vi "RatTracker.vi"() -> ()   [LabVIEW 2014]
doc: "Capture_32bit nimmt kontinuierlich Bilder von der Kamera auf und zeigt diese an."
panel:
  out "Elapsed Time (s)":dbl
  out "Rat Name":string
  out "Dropped Frame Count":dbl
  out "AVI Frame Number":dbl
  out "Codec Names":string[](array[string])
  out "error out":errorcluster caption="error"
  out "Video":T1(plugin-control)
  in  "Camera ID":u32
  out "Height":i32=480
  out "Width":i32=640
  out "Bits/Pixel":i32=8
  out "FPS":dbl=6.258409738085552
  in  "Blue Gain":i32(slide) min=0 max=100 scale=0.0..100.0
  in  "Red Gain":i32(slide) min=0 max=100 scale=0.0..100.0
  in  "Green Gain":i32(slide) min=0 max=100 scale=0.0..100.0
  in  "Exposure time":dbl(slide)=33.21525 min=0.0286 max=15.987400000000001 step=0.0286 scale=0.0286..15.987400000000001 scale format="%#.3g"
  in  "Auto Shutter":bool
  in  "Auto Whitebalance":bool
  in  "Color Correction":bool
  in  "Frame rate":dbl(slide)=59.79798117517122 min=1.0506320602474448 max=63.11378152533386 step=2.86e-05 scale=1.0506320602474448..63.11378152533386 scale format="%^#_3g"
  in  "Pixel clock":i32(slide)=29 min=5 max=40 scale=5.0..40.0
  in  "Edge Filter":i32(ring)=2 items=["High"=1, "Low"=2]
  in  "Edge Filter Enable / Disable":bool
  in  "Blacklevel Offset":i32(slide) min=0 max=255 scale=0.0..255.0
  in  "Blacklevel Compensation":bool
  in  "Hotpixel correction":bool
  in  "Master Gain":i32(slide)=90 min=0 max=100 scale=0.0..100.0
  in  "Autogain":bool
  in  "Stop":bool
  # "Hello! Press the white arrow in the top-left to start recording."
  # "NOTE: When ending the program, you must use the STOP button below! Otherwise, you will have to restart the computer in order to use the camera again!"
  # "Stop Program here"
  # "Settings"
  # "Image information"
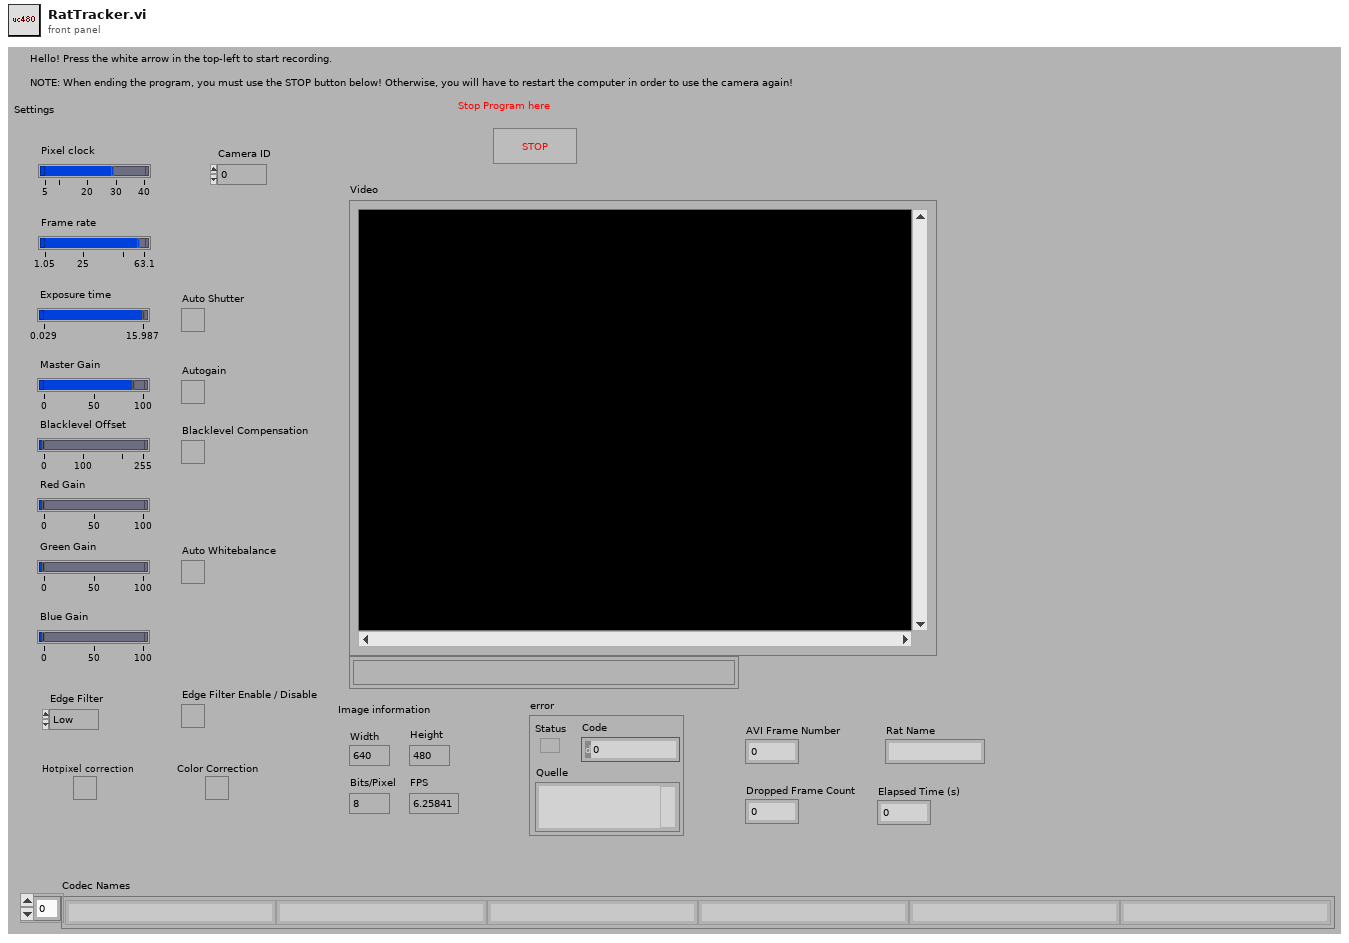
[diagram p1: front panel]
types:
  T1 = typedef "IMAQ Image.ctl" = refnum<image>
  T2 = typedef "IMAQ AVI2 Refnum.ctl" = refnum<k20>
  T3 = cluster{"Height":i32, "Width":i32, "Bits/Pixel":i32}
  T4 = cluster{"Codec Names[0]":string, "Codec Names[1]":string, "Codec Names[2]":string, "Codec Names[3]":string, "Codec Names[4]":string, "Codec Names[5]":string, "Codec Names[6]":string, "Codec Names[7]":string, "Codec Names[8]":string}
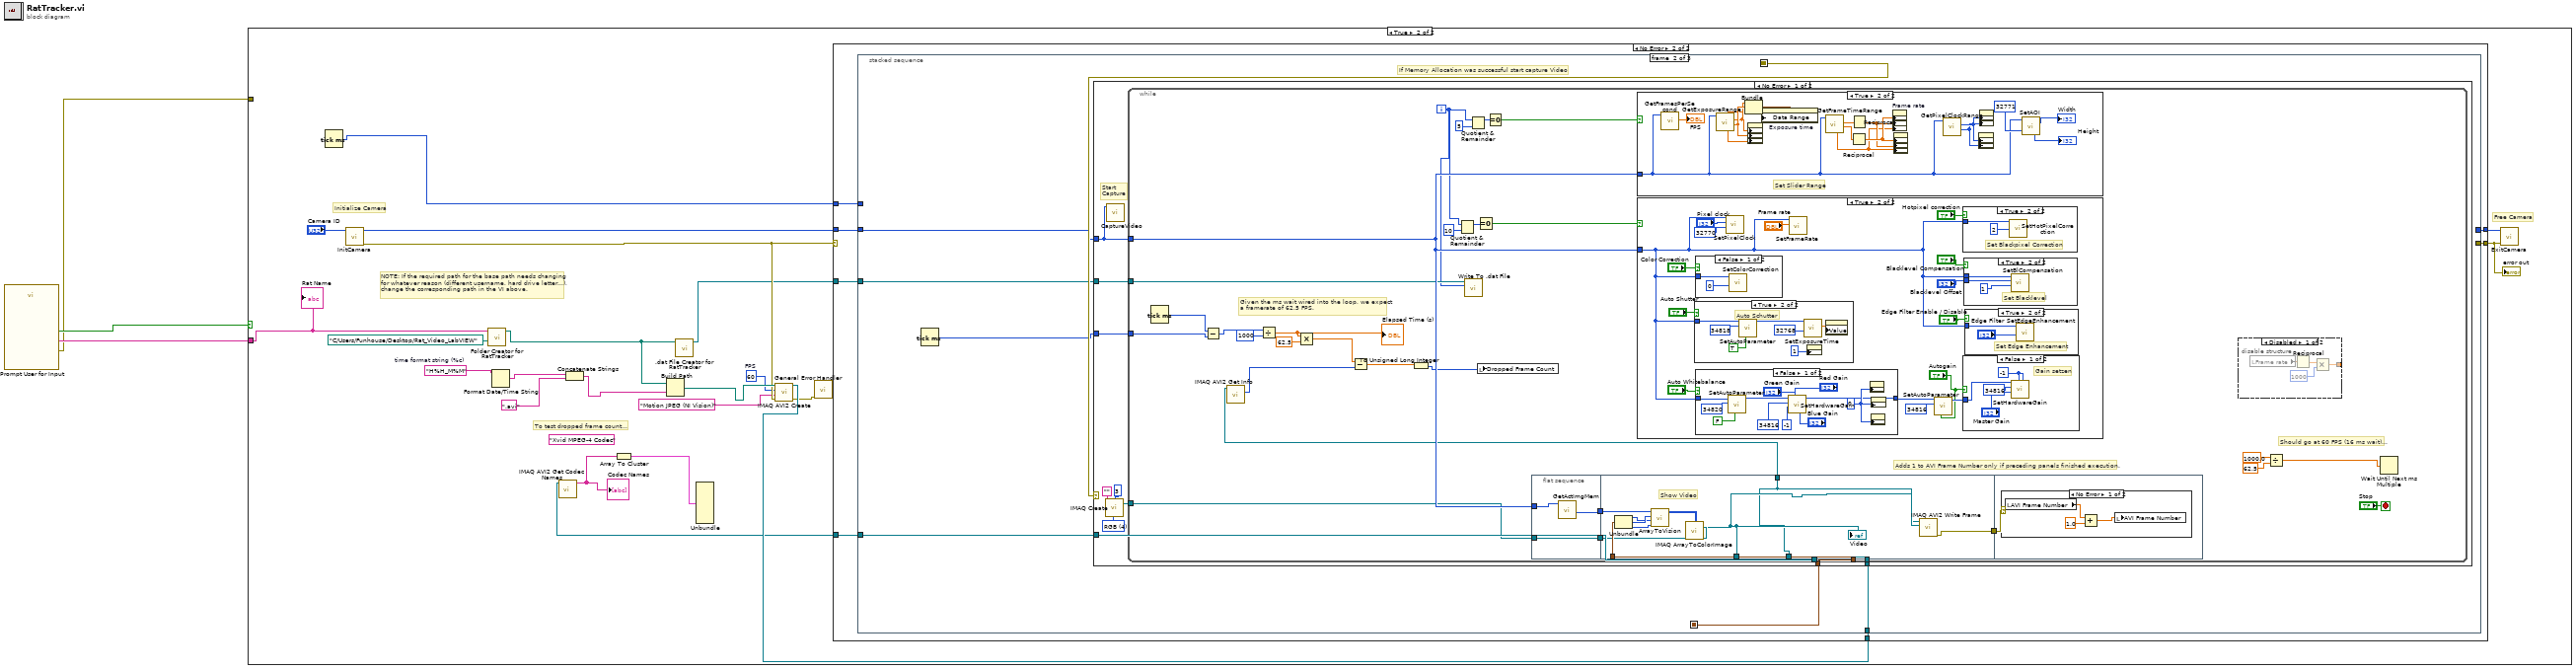
[diagram p0: block diagram]
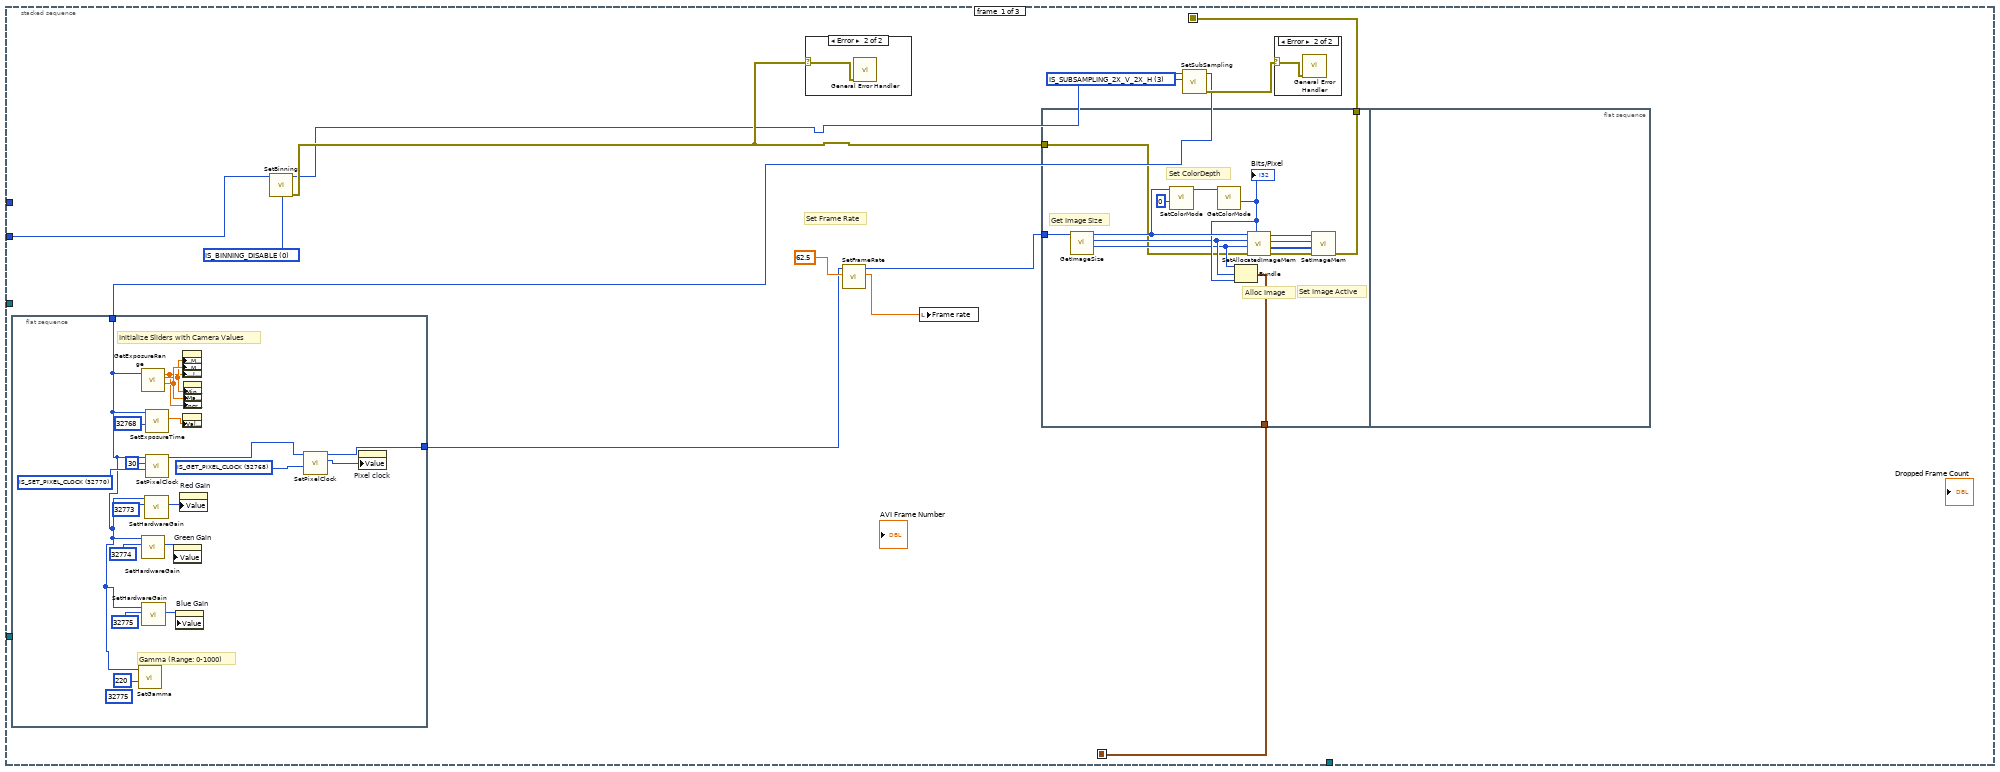
[diagram p4: hidden frame]
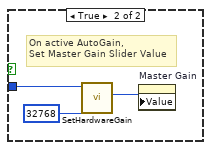
[diagram p9: hidden frame]
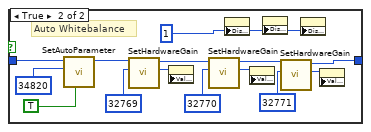
[diagram p10: hidden frame]
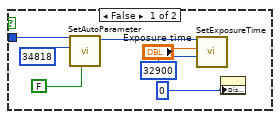
[diagram p11: hidden frame]
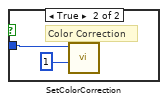
[diagram p12: hidden frame]
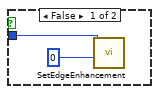
[diagram p13: hidden frame]
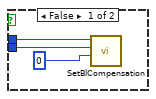
[diagram p14: hidden frame]
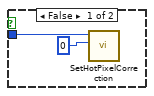
[diagram p15: hidden frame]
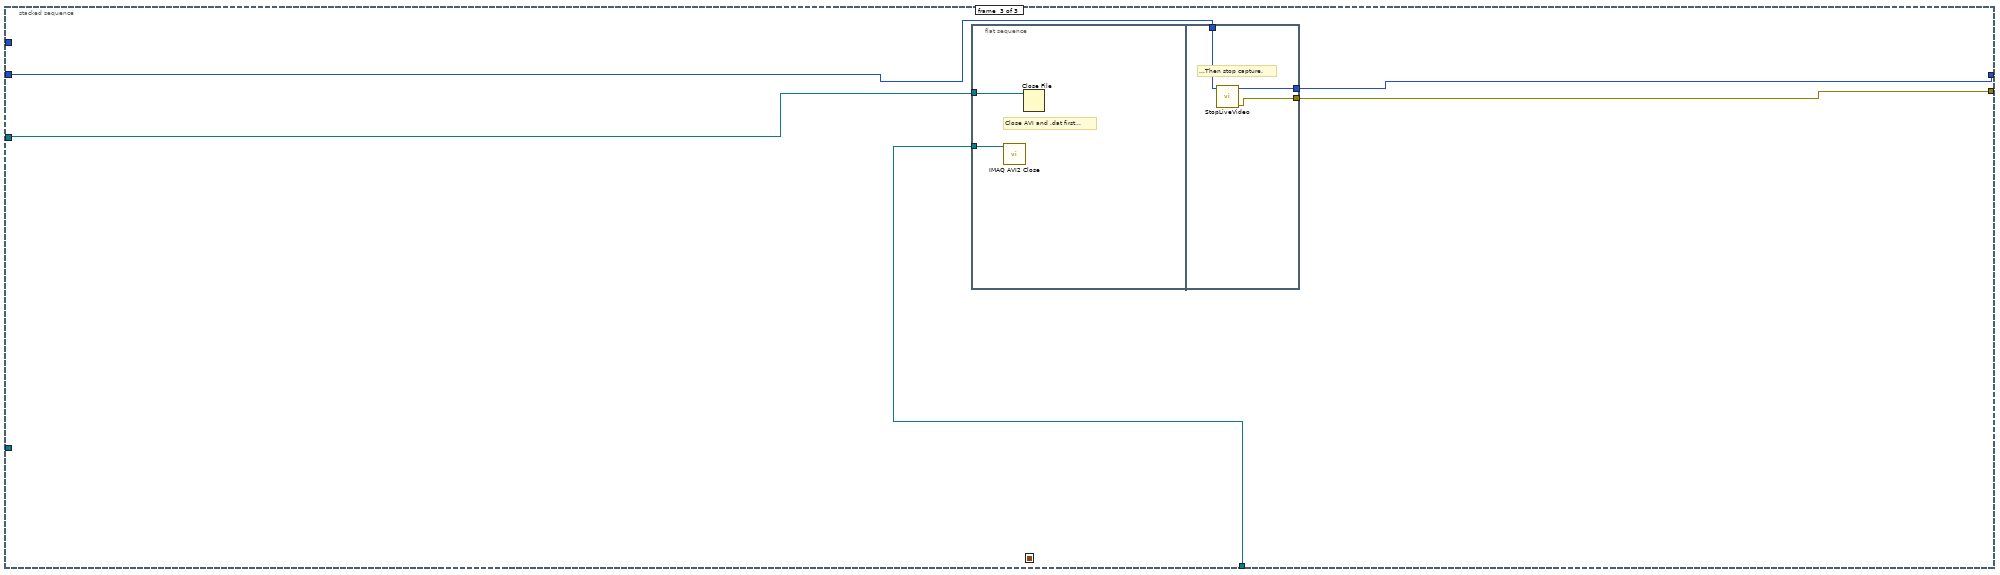
[diagram p19: hidden frame]
diagram:
  n1 = call "Prompt User for Input"() -> ("Name"=w2:string, "OK"=w3:bool, "error out"=w1:errorcluster)  [unwired: 17 in]
  n2 = case shown="True" w3 {
    tunnel: w2 -> [_ w15]
    tunnel: w1 -> [_ _]
    frame False {
    }
    frame True {
      (unwired) "Xvid MPEG-4 Codec"
      w7 = u32 60  # FPS
      w19 = "H%H_M%M"  # time format string (%c)
      # "To test dropped frame count..."
      # "NOTE: If the required path for the base path needs changing\nfor whatever reason (different username, hard drive letter...),\nchange the corresponding path in the VI above."
      # "Free Camera"
      # "Initialize Camera"
      n3 = Tick Count (ms)() -> (millisecond timer value=w5:u32)
      n4 = call "InitCamera.vi"("Camera ID"="Camera ID") -> ("error out"=w12:errorcluster, "Camera Handle Out"=w24:u32)  [unwired: 9 in]
      n5 = call "Folder Creator for RatTracker.vi"("Base Path"=path "C:/Users/Funhouse/Desktop/Rat_Video_LabVIEW" ("Base Path for File"), "Rat Name"=w15) -> ("Path of Folder with .avi and .dat"=w16:path)  [unwired: 9 in]
      n6 = Format Date/Time String(time format string (%c)=w19) -> (date/time string=w20:string)  [unwired: 2 in]
      n7 = Concatenate Strings(w20, ".avi") -> (w17:string)
      n8 = Build Path(base path=w16, name or relative path=w17) -> (appended path=w14:path)
      n9 = call ".dat File Creator for RatTracker.vi"("Path of Folder with .avi and .dat"=w16) -> ("Reference to .dat File"=w8:refnum<file>)  [unwired: 10 in]
      n10 = call "IMAQ AVI2 Create"("error in (no error)"=w12, "Codec"="Motion JPEG (NI Vision)", "Frames Per Second"=w7, "AVI Path"=w14) -> ("error out"=w6:errorcluster, "AVI Refnum"=w13:T2)  [unwired: 6 in]
      n11 = call <vilib>:"General Error Handler.vi"("error in (no error)"=w6) -> ()  [unwired: 10 in, 5 out]
      n12 = case shown="No Error" w12 {
        selector: w12 -> [w26 _]
        tunnel: [w27 w34] -> w25
        tunnel: w24 -> [w27 w33]
        tunnel: [w26 w32] -> w22
        tunnel: w13 -> [_ w31]
        tunnel: [_ w30] -> w11
        tunnel: w8 -> [_ w29]
        tunnel: w5 -> [_ w28]
        frame Error {
        }
        frame No Error {
          n13 = stacked-sequence {
            seq-local: [w46 _ _] -> [_ w89 _]
            seq-local: [w47 _ _] -> [_ w88 _]
            tunnel: w33 -> [w45 w87 w249]
            tunnel: [_ _ w248] -> w34
            tunnel: [_ _ w250] -> w32
            tunnel: w31 -> [_ w86 w251]
            tunnel: [_ w85 _] -> w30
            tunnel: w29 -> [_ w84 w247]
            tunnel: w28 -> [_ _ _]
            frame #0 {
              w40 = 3 items=["IS_SUBSAMPLING_DISABLE"=0, "IS_SUBSAMPLING_2X_V"=1, "IS_SUBSAMPLING_2X_H"=2, "IS_SUBSAMPLING_4X_V"=4, "IS_SUBSAMPLING_4X_H"=8, "IS_SUBSAMPLING_2X_V_2X_H"=3, "IS_SUBSAMPLING_4X_V_2X_H"=6, "IS_SUBSAMPLING_2X_V_4X_H"=9, "IS_SUBSAMPLING_4X_V_4X_H"=12, "IS_GET_SUBSAMPLING"=32768, "IS_GET_SUPPORTED_SUBSAMPLING"=32769] ("Mode")
              w44 = 0 items=["IS_BINNING_DISABLE"=0, "IS_BINNING_2X_V"=1, "IS_BINNING_2X_H"=2, "IS_BINNING_4X_V"=4, "IS_BINNING_4X_H"=8, "IS_BINNING_2X_V_2X_H"=3, "IS_BINNING_2X_V_4X_H"=9, "IS_BINNING_4X_V_2X_H"=6, "IS_BINNING_4X_V_4X_H"=12, "IS_GET_BINNING"=32768, "IS_GET_SUPPORTED_BINNING"=32769] ("Mode")
              # "Set Frame Rate"
              n14 = flat-sequence {
                tunnel: w37 -> [w63]
                tunnel: [w65] -> w36
                frame #0 {
                  (unwired) 32775
                  w68 = 32768 items=["IS_GET_PIXEL_CLOCK"=32768, "IS_GET_DEFAULT_PCLK"=32769, "IS_SET_PIXEL_CLOCK"=32770] ("Mode")
                  w69 = 32770 items=["IS_GET_PIXEL_CLOCK"=32768, "IS_GET_DEFAULT_PCLK"=32769, "IS_SET_PIXEL_CLOCK"=32770] ("Mode")
                  # "Gamma (Range: 0-1000)"
                  # "Initialize Sliders with Camera Values"
                  n15 = call "SetGamma.vi"("Gamma"=220, "Camera Handle In"=w63) -> ()  [unwired: 8 in, 2 out]
                  n16 = call "GetExposureRange.vi"("Camera Handle In"=w63) -> ("max"=w80:dbl, "min"=w79:dbl, "intervall"=w78:dbl)  [unwired: 6 in, 2 out]
                  n17 = call "SetHardwareGain.vi"("Mode"=32774, "Camera Handle In"=w63) -> ("Value"=w73:i32)  [unwired: 7 in, 2 out]
                  n18 = call "SetHardwareGain.vi"("Mode"=32775, "Camera Handle In"=w63) -> ("Value"=w71:i32)  [unwired: 7 in, 2 out]
                  n19 = call "SetHardwareGain.vi"("Mode"=32773, "Camera Handle In"=w63) -> ("Value"=w75:i32)  [unwired: 7 in, 2 out]
                  n20 = call "SetExposureTime.vi"("Mode"=u16 32768, "Camera Handle In"=w63) -> ("new exposure time"=w76:dbl)  [unwired: 7 in, 2 out]
                  n21 = call "SetPixelClock.vi"("Mode"=w69, "Pixel Clock"=30, "Camera Handle In"=w63) -> ("Camera Handle Out"=w67:u32)  [unwired: 6 in, 2 out]
                  n22 = property on="Green Gain" class="Slide (strict)"("Value"=w73) -> ()  [unwired: 2 in, 2 out]
                  n23 = property on="Blue Gain" class="Slide (strict)"("Value"=w71) -> ()  [unwired: 2 in, 2 out]
                  n24 = property on="Red Gain" class="Slide (strict)"("Value"=w75) -> ()  [unwired: 2 in, 2 out]
                  n25 = property on="Exposure time" class="Schieberegler (strikt)"("Scale.Minimum"=w79, "Scale.Maximum"=w80, "Scale.Increment"=w78) -> ()  [unwired: 2 in, 2 out]
                  n26 = property on="Exposure time" class="Schieberegler (strikt)"("Value"=w76) -> ()  [unwired: 2 in, 2 out]
                  n27 = property on="Exposure time" class="Schieberegler (strikt)"("Minimum"=w79, "Maximum"=w80, "Increment"=w78) -> ()  [unwired: 2 in, 2 out]
                  n28 = call "SetPixelClock.vi"("Mode"=w68, "Camera Handle In"=w67) -> ("Value"=w66:i32, "Camera Handle Out"=w65:u32)  [unwired: 7 in, 1 out]
                  n29 = property on="Pixel clock" class="Slide (strict)"("Value"=w66) -> ()  [unwired: 2 in, 2 out]
                }
              }
              n30 = call "SetBinning.vi"("Mode"=w44, "Camera Handle In"=w45) -> ("error out"=w43:errorcluster, "Camera Handle Out"=w42:u32)  [unwired: 7 in, 1 out]
              n31 = case shown="Error" w43 {
                selector: w43 -> [_ w82]
                frame No Error {
                }
                frame Error {
                  n32 = call <vilib>:"General Error Handler.vi"("error in (no error)"=w82) -> ()  [unwired: 10 in, 5 out]
                }
              }
              n33 = call "SetFrameRate.vi"("FPS"=62.5, "Camera Handle In"=w36) -> ("new FPS"=w35:dbl, "Camera Handle Out"=w39:u32)  [unwired: 7 in, 1 out]
              n34 = local write "Frame rate"(w35) -> ()
              n35 = flat-sequence {
                tunnel: [w58] -> w47
                tunnel: [w56] -> w46
                tunnel: w43 -> [w49]
                tunnel: w39 -> [w48]
                frame #0 {
                  # "Set Image Active"
                  # "Alloc Image"
                  # "Set ColorDepth"
                  # "Get Image Size"
                  n36 = call "GetImageSize.vi"("Camera Handle In"=w48) -> ("Height"=w50:i32, "Width"=w51:i32, "Camera Handle Out"=w57:u32)  [unwired: 8 in]
                  n37 = call "SetColorMode.vi"("Mode"=0, "Camera Handle In"=w57) -> ("Camera Handle Out"=w53:u32)  [unwired: 8 in, 1 out]
                  n38 = call "GetColorMode.vi"("Camera Handle In"=w53) -> ("Bits/Pixel"=w52:i32)  [unwired: 8 in, 2 out]
                  "Bits/Pixel" <- w52
                  n39 = Bundle("Height"=w50, "Width"=w51, "Bits/Pixel"=w52) -> (w56:T3)  [unwired: 1 in]
                  n40 = call "SetAllocatedImageMem.vi"("BitsPixel"=w52, "error in"=w49, "Height"=w50, "Width"=w51, "Camera Handle In"=w57) -> ("error out"=w55:errorcluster, "Image Memory Out"=w59:u8[], "Memory ID Out"=w60:i32, "Camera Handle Out"=w61:u32)  [unwired: 2 in, 1 out]
                  n41 = call "SetImageMem.vi"("error in"=w55, "Image Memory In"=w59, "Memory ID In"=w60, "Camera Handle In"=w61) -> ("error out"=w58:errorcluster)  [unwired: 4 in, 3 out]
                }
                frame #1 {
                }
              }
              n42 = call "SetSubSampling.vi"("Mode"=w40, "Camera Handle In"=w42) -> ("error out"=w41:errorcluster, "Camera Handle Out"=w37:u32)  [unwired: 7 in, 1 out]
              n43 = case shown="Error" w41 {
                selector: w41 -> [_ w81]
                frame No Error {
                }
                frame Error {
                  n44 = call <vilib>:"General Error Handler.vi"("error in (no error)"=w81) -> ()  [unwired: 10 in, 5 out]
                }
              }
            }
            frame #1 {
              # "If Memory Allocation was successful start capture Video"
              n45 = Tick Count (ms)() -> (millisecond timer value=w83:u32)
              n46 = case shown="No Error" w88 {
                tunnel: w87 -> [w98 _]
                tunnel: w89 -> [w99 _]
                tunnel: w86 -> [w93 _]
                tunnel: [w92 _] -> w85
                tunnel: w84 -> [w91 _]
                tunnel: w83 -> [w90 _]
                frame No Error {
                  w96 = u32 4 items=["8 bits", "16 bits", "Float", "Complex", "RGB", "HSL"] ("Image Type")
                  # "Start\nCapture"
                  n47 = call "IMAQ Create"("Border Size"=3, "Image Name"="", "Image Type"=w96) -> ("New Image"=w94:T1)  [unwired: 2 in, 1 out]
                  n48 = call "CaptureVideo.vi"("Camera Handle In"=w98) -> ()  [unwired: 9 in, 2 out]
                  n49 = while {
                    tunnel: w99 -> [w129]
                    tunnel: w98 -> [w121]
                    tunnel: w94 -> [w119]
                    tunnel: w93 -> [w118]
                    tunnel: [w117] -> w92
                    tunnel: w91 -> [w116]
                    tunnel: w90 -> [w112]
                    i -> [w115]
                    stop <- "Stop" stop-if-true
                    # "Given the ms wait wired into the loop, we expect\na framerate of 62.5 FPS."
                    # "Should go at 60 FPS (16 ms wait)..."
                    # "Adds 1 to AVI Frame Number only if preceding panels finished execution."
                    n50 = Tick Count (ms)() -> (millisecond timer value=w111:u32)
                    n51 = Subtract(x=w111, y=w112) -> (x-y=w110:u32)
                    n52 = call "IMAQ AVI2 Get Info"("AVI Refnum"=w113) -> ("Number of Frames"=w105:u32)  [unwired: 6 in, 4 out]
                    n53 = Divide(x=w110, y=u32 1000) -> (x/y=w108:dbl)
                    "Elapsed Time (s)" <- w108
                    n54 = Multiply(x=w108, y=62.5) -> (x*y=w106:dbl)
                    n55 = Subtract(x=w106, y=w105) -> (x-y=w101:dbl)
                    n56 = To Unsigned Long Integer(number=w101) -> (unsigned 32bit integer=w100:u32)
                    n57 = Quotient & Remainder(x=w115, y=10) -> (x-y*floor(x/y)=w124:i32)  [unwired: 1 out]
                    n58 = call "Write To .dat File.vi"("Frame Number"=w115, ".dat File"=w116) -> ()  [unwired: 9 in, 1 out]
                    n59 = Quotient & Remainder(x=w115, y=5) -> (x-y*floor(x/y)=w127:i32)  [unwired: 1 out]
                    n60 = Equal To 0?(x=w124) -> (x = 0?=w122:bool)
                    n61 = local write "Dropped Frame Count"(w100) -> ()
                    n62 = Equal To 0?(x=w127) -> (x = 0?=w126:bool)
                    n63 = flat-sequence {
                      tunnel: [w230] -> w130
                      tunnel: w121 -> [w231]
                      tunnel: [w232] -> w120
                      tunnel: w119 -> [w232]
                      tunnel: w130 -> [w241]
                      tunnel: w129 -> [w242]
                      tunnel: w120 -> [w237]
                      tunnel: w118 -> [w233]
                      tunnel: [w235] -> w117
                      tunnel: [w234] -> w114
                      tunnel: [w233] -> w113
                      tunnel: w114 -> [w243]
                      frame #0 {
                        n64 = call "GetActImgMem.vi"("Camera Handle In"=w231) -> ("Image Memory Out"=w230:u8[])  [unwired: 7 in, 3 out]
                      }
                      frame #1 {
                        # "Show Video"
                        n65 = Unbundle(w242) -> ("Height"=w238:i32, "Width"=w240:i32, "Bits/Pixel"=w239:i32)
                        n66 = call "ArrayToVision.vi"("Bits/Pixel"=w239, "Height"=w238, "Width"=w240, "InArray"=w241) -> ("OutArray"=w236:u32[][])  [unwired: 7 in]
                        n67 = call "IMAQ ArrayToColorImage"("Image Pixels (U32)"=w236, "Image"=w237) -> ("Image Out"=w235:T1)  [unwired: 3 in, 1 out]
                        "Video" <- w235
                        n68 = call "IMAQ AVI2 Write Frame"("Image"=w235, "AVI Refnum"=w233) -> ("error out"=w234:errorcluster)  [unwired: 7 in, 2 out]
                      }
                      frame #2 {
                        n69 = case shown="No Error" w243 {
                          frame No Error {
                            n70 = local read "AVI Frame Number"() -> (w246:dbl)
                            n71 = Add(x=w246, y=1.0) -> (x+y=w244:dbl)
                            n72 = local write "AVI Frame Number"(w244) -> ()
                          }
                          frame Error {
                          }
                        }
                      }
                    }
                    n73 = case shown="True" w126 {
                      tunnel: w121 -> [_ w217]
                      frame False {
                      }
                      frame True {
                        # "Set Slider Range"
                        n74 = call "GetFramesPerSecond.vi"("Camera Handle In"=w217) -> ("FPS"=→"FPS":dbl)  [unwired: 8 in, 2 out]
                        n75 = call "GetExposureRange.vi"("Camera Handle In"=w217) -> ("max"=w216:dbl, "min"=w215:dbl, "intervall"=w214:dbl)  [unwired: 6 in, 2 out]
                        n76 = Bundle("min"=w215, "max"=w216, "intervall"=w214) -> (w227:cluster{"min":dbl, "max":dbl, "intervall":dbl})  [unwired: 1 in]
                        n77 = property on="Exposure time" class="Schieberegler (strikt)"("Scale.Minimum"=w215, "Scale.Maximum"=w216, "Scale.Increment"=w214) -> ()  [unwired: 2 in, 2 out]
                        n78 = property on="Exposure time" class="Slide (strict)"("Data Range"=w227) -> ()  [unwired: 2 in, 2 out]
                        n79 = call "GetFrameTimeRange.vi"("Camera Handle In"=w217) -> ("max"=w219:dbl, "min"=w218:dbl, "interval"=w220:dbl)  [unwired: 6 in, 2 out]
                        n80 = Reciprocal(x=w219) -> (1/x=w229:dbl)
                        n81 = Reciprocal(x=w218) -> (1/x=w228:dbl)
                        n82 = property on="Frame rate" class="Schieberegler (strikt)"("Minimum"=w229, "Maximum"=w228, "Increment"=w220) -> ()  [unwired: 2 in, 2 out]
                        n83 = property on="Frame rate" class="Schieberegler (strikt)"("Scale.Minimum"=w229, "Scale.Maximum"=w228, "Scale.Increment"=w220) -> ()  [unwired: 2 in, 2 out]
                        n84 = call "GetPixelClockRange.vi"("Camera Handle In"=w217) -> ("Max"=w221:i32, "Min"=w222:i32)  [unwired: 7 in, 2 out]
                        n85 = property on="Pixel clock" class="Schieberegler (strikt)"("Scale.Minimum"=w222, "Scale.Maximum"=w221) -> ()  [unwired: 2 in, 2 out]
                        n86 = property on="Pixel clock" class="Schieberegler (strikt)"("Minimum"=w222, "Maximum"=w221) -> ()  [unwired: 2 in, 2 out]
                        n87 = call "SetAOI.vi"("Camera Handle In"=w217, "Mode"=32771) -> ("Width Out"=→"Width":i32, "Height Out"=→"Height":i32)  [unwired: 8 in, 4 out]
                      }
                    }
                    n88 = case shown="True" w122 {
                      tunnel: w121 -> [_ w140]
                      frame False {
                      }
                      frame True {
                        n89 = case shown="True" "Auto Shutter" {
                          tunnel: w140 -> [w187 w194]
                          frame False {
                            n90 = call "SetAutoParameter.vi"("enable"=FALSE, "Param"=34818, "Camera Handle In"=w187) -> ("Camera Handle Out"=w184:u32)  [unwired: 6 in, 2 out]
                            n91 = call "SetExposureTime.vi"("Mode"=u16 32900, "Exposure Time"="Exposure time", "Camera Handle In"=w184) -> ()  [unwired: 6 in, 3 out]
                            n92 = property on="Exposure time" class="Schieberegler (strikt)"("Disabled"=u8 0) -> ()  [unwired: 2 in, 2 out]
                          }
                          frame True {
                            # "Auto Schutter"
                            n93 = call "SetAutoParameter.vi"("enable"=TRUE, "Param"=34818, "Camera Handle In"=w194) -> ("Camera Handle Out"=w192:u32)  [unwired: 6 in, 2 out]
                            n94 = call "SetExposureTime.vi"("Mode"=u16 32768, "Camera Handle In"=w192) -> ("new exposure time"=w189:dbl)  [unwired: 7 in, 2 out]
                            n95 = property on="Exposure time" class="Schieberegler (strikt)"("Disabled"=u8 1) -> ()  [unwired: 2 in, 2 out]
                            n96 = property on="Exposure time" class="Slide (strict)"("Value"=w189) -> ()  [unwired: 2 in, 2 out]
                          }
                        }
                        n97 = case shown="False" "Color Correction" {
                          tunnel: w140 -> [w197 w199]
                          frame False {
                            n98 = call "SetColorCorrection.vi"("Mode"=0, "Camera Handle In"=w197) -> ()  [unwired: 8 in, 2 out]
                          }
                          frame True {
                            # "Color Correction"
                            n99 = call "SetColorCorrection.vi"("Mode"=1, "Camera Handle In"=w199) -> ()  [unwired: 8 in, 2 out]
                          }
                        }
                        n100 = case shown="False" "Auto Whitebalance" {
                          tunnel: w140 -> [w166 w180]
                          tunnel: [w163 w173] -> w137
                          frame False {
                            w167 = u8 0
                            n101 = call "SetAutoParameter.vi"("enable"=FALSE, "Param"=34820, "Camera Handle In"=w166) -> ("Camera Handle Out"=w162:u32)  [unwired: 6 in, 2 out]
                            n102 = call "SetHardwareGain.vi"("Blue"="Blue Gain", "Green"="Green Gain", "Red"="Red Gain", "Master Gain"=-1, "Mode"=34816, "Camera Handle In"=w162) -> ("Camera Handle Out"=w163:u32)  [unwired: 3 in, 2 out]
                            n103 = property on="Blue Gain" class="Schieberegler (strikt)"("Disabled"=w167) -> ()  [unwired: 2 in, 2 out]
                            n104 = property on="Green Gain" class="Schieberegler (strikt)"("Disabled"=w167) -> ()  [unwired: 2 in, 2 out]
                            n105 = property on="Red Gain" class="Schieberegler (strikt)"("Disabled"=w167) -> ()  [unwired: 2 in, 2 out]
                          }
                          frame True {
                            w181 = u8 1
                            # "Auto Whitebalance"
                            n106 = call "SetAutoParameter.vi"("enable"=TRUE, "Param"=34820, "Camera Handle In"=w180) -> ("Camera Handle Out"=w176:u32)  [unwired: 6 in, 2 out]
                            n107 = call "SetHardwareGain.vi"("Mode"=32769, "Camera Handle In"=w176) -> ("Value"=w177:i32, "Camera Handle Out"=w175:u32)  [unwired: 7 in, 1 out]
                            n108 = property on="Red Gain" class="Schieberegler (strikt)"("Value"=w177) -> ()  [unwired: 2 in, 2 out]
                            n109 = call "SetHardwareGain.vi"("Mode"=32770, "Camera Handle In"=w175) -> ("Value"=w172:i32, "Camera Handle Out"=w174:u32)  [unwired: 7 in, 1 out]
                            n110 = property on="Red Gain" class="Schieberegler (strikt)"("Disabled"=w181) -> ()  [unwired: 2 in, 2 out]
                            n111 = property on="Green Gain" class="Schieberegler (strikt)"("Value"=w172) -> ()  [unwired: 2 in, 2 out]
                            n112 = property on="Green Gain" class="Schieberegler (strikt)"("Disabled"=w181) -> ()  [unwired: 2 in, 2 out]
                            n113 = call "SetHardwareGain.vi"("Mode"=32771, "Camera Handle In"=w174) -> ("Value"=w171:i32, "Camera Handle Out"=w173:u32)  [unwired: 7 in, 1 out]
                            n114 = property on="Blue Gain" class="Schieberegler (strikt)"("Disabled"=w181) -> ()  [unwired: 2 in, 2 out]
                            n115 = property on="Blue Gain" class="Schieberegler (strikt)"("Value"=w171) -> ()  [unwired: 2 in, 2 out]
                          }
                        }
                        n116 = call "SetPixelClock.vi"("Mode"=32770, "Pixel Clock"="Pixel clock", "Camera Handle In"=w140) -> ()  [unwired: 6 in, 3 out]
                        n117 = call "SetFrameRate.vi"("FPS"="Frame rate", "Camera Handle In"=w140) -> ()  [unwired: 7 in, 3 out]
                        n118 = call "SetAutoParameter.vi"("enable"="Autogain", "Param"=34816, "Camera Handle In"=w137) -> ("Camera Handle Out"=w138:u32)  [unwired: 6 in, 2 out]
                        n119 = case shown="True" "Hotpixel correction" {
                          tunnel: w140 -> [w211 w213]
                          frame False {
                            n120 = call "SetHotPixelCorrection.vi"("Mode"=0, "Camera Handle In"=w211) -> ()  [unwired: 7 in, 3 out]
                          }
                          frame True {
                            # "Set Blackpixel Correction"
                            n121 = call "SetHotPixelCorrection.vi"("Mode"=2, "Camera Handle In"=w213) -> ()  [unwired: 7 in, 3 out]
                          }
                        }
                        n122 = case shown="False" "Autogain" {
                          tunnel: w138 -> [w153 w156]
                          frame False {
                            w150 = -1
                            # "Gain setzen"
                            n123 = call "SetHardwareGain.vi"("Blue"=w150, "Green"=w150, "Red"=w150, "Master Gain"="Master Gain", "Mode"=34816, "Camera Handle In"=w153) -> ()  [unwired: 3 in, 3 out]
                          }
                          frame True {
                            # "On active AutoGain,\nSet Master Gain Slider Value"
                            n124 = call "SetHardwareGain.vi"("Mode"=32768, "Camera Handle In"=w156) -> ("Value"=w154:i32)  [unwired: 7 in, 2 out]
                            n125 = property on="Master Gain" class="Slide (strict)"("Value"=w154) -> ()  [unwired: 2 in, 2 out]
                          }
                        }
                        n126 = case shown="True" "Blacklevel Compensation" {
                          tunnel: w140 -> [w206 w209]
                          tunnel: "Blacklevel Offset" -> [w205 w208]
                          frame False {
                            n127 = call "SetBlCompensation.vi"("Mode"=0, "offset"=w205, "Camera Handle In"=w206) -> ()  [unwired: 6 in, 3 out]
                          }
                          frame True {
                            # "Set Blacklevel"
                            n128 = call "SetBlCompensation.vi"("Mode"=1, "offset"=w208, "Camera Handle In"=w209) -> ()  [unwired: 6 in, 3 out]
                          }
                        }
                        n129 = case shown="True" "Edge Filter Enable / Disable" {
                          tunnel: w140 -> [w201 w203]
                          frame False {
                            n130 = call "SetEdgeEnhancement.vi"("Mode"=0, "Camera Handle In"=w201) -> ()  [unwired: 8 in, 2 out]
                          }
                          frame True {
                            # "Set Edge Enhancement"
                            n131 = call "SetEdgeEnhancement.vi"("Mode"="Edge Filter", "Camera Handle In"=w203) -> ()  [unwired: 8 in, 2 out]
                          }
                        }
                      }
                    }
                    n132 = disable-structure shown="Disabled" {
                      disable-tunnel: [w132 _] -> _
                      frame Disabled {
                        n133 = local read "Frame rate"() -> (w134:dbl)
                        n134 = Reciprocal(x=w134) -> (1/x=w133:dbl)
                        n135 = Multiply(x=w133, y=1000) -> (x*y=w132:dbl)
                      }
                      frame Enabled {
                      }
                    }
                    n136 = Divide(x=1000.0, y=62.5) -> (x/y=w102:dbl)
                    n137 = Wait Until Next ms Multiple(millisecond multiple=w102) -> ()  [unwired: 1 out]
                  }
                }
                frame Error {
                }
              }
            }
            frame #2 {
              n138 = flat-sequence {
                tunnel: w251 -> [w253]
                tunnel: w247 -> [w252]
                tunnel: [w256] -> w250
                tunnel: w249 -> [w255]
                tunnel: [w254] -> w248
                frame #0 {
                  # "Close AVI and .dat first..."
                  n139 = call "IMAQ AVI2 Close"("AVI Refnum"=w253) -> ()  [unwired: 10 in, 1 out]
                  n140 = Close File(refnum=w252) -> ()  [unwired: 1 in, 2 out]
                }
                frame #1 {
                  # "...Then stop capture."
                  n141 = call "StopLiveVideo.vi"("Camera Handle In"=w255) -> ("error out"=w256:errorcluster, "Camera Handle Out"=w254:u32)  [unwired: 9 in]
                }
              }
            }
          }
        }
      }
      "error out" <- w22
      n142 = call "IMAQ AVI2 Get Codec Names"("Image"=w11) -> ("Codec Names"=w10:string[])  [unwired: 9 in, 1 out]
      "Codec Names" <- w10
      n143 = Array To Cluster(array=w10) -> (cluster=w9:T4)
      n144 = Unbundle "Unbundle"(w9) -> ()  [unwired: 9 out]
      n145 = call "ExitCamera.vi"("error in"=w22, "Camera Handle In"=w25) -> ()  [unwired: 9 in, 1 out]
      "Rat Name" <- w15
    }
  }
